vi "SysDef.Node.Info.vi"(8 "error in (no error)":errorcluster, 11 "nodeID":u64) -> (0 "error out":errorcluster, 1 "Item Info":T1, 3 "nodeID out":u64, 4 "Found?":bool)   [LabVIEW 2019, in "Advanced System Definition.lvlib"]
uses:
  Advanced System Definition.lvlib
  _Types/TreeItem.Info.ctl
  <vilib>/NI VeriStand/Custom Device API/Custom Device Channel.ctl
  <vilib>/NI VeriStand/Custom Device API/Custom Device Channel Type.ctl
  <vilib>/NI VeriStand/Custom Device API/Custom Device Waveform.ctl
  <vilib>/NI VeriStand/Custom Device API/Custom Device Waveform DataType.ctl
  NationalInstruments.VeriStand.SystemDefinitionAPI
  <vilib>/NI VeriStand/Custom Device API/Custom Device API.lvlib
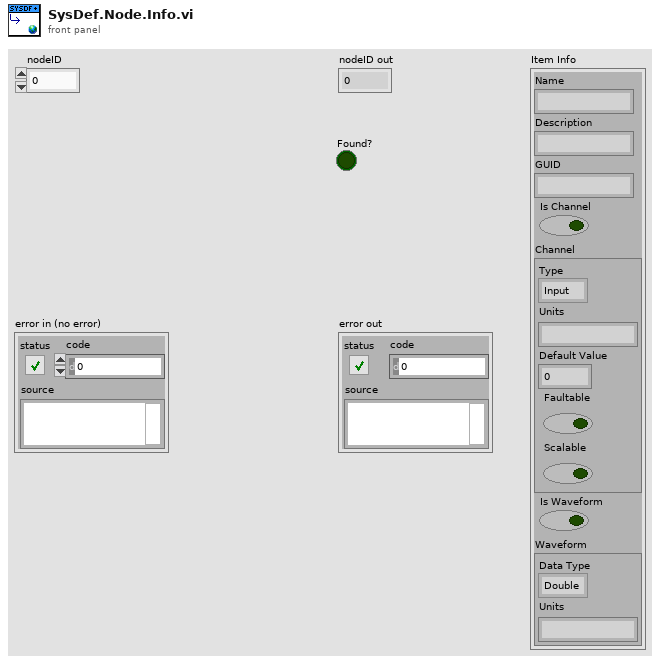
[diagram p1: front panel]
types:
  T1 = typedef "Advanced System Definition.lvlib/TreeItem.Info.ctl" = cluster{"Name":string, "Description":string, "GUID":string, "Is Channel":bool, "Channel":T2, "Is Waveform":bool, "Waveform":T4}
  T2 = typedef "Custom Device API.lvlib/Custom Device Channel.ctl" = cluster{"Type":T3, "Units":string, "Default Value":dbl, "Faultable":bool, "Scalable":bool}
  T3 = typedef "Custom Device API.lvlib/Custom Device Channel Type.ctl" = enum16{"Input", "Output"}
  T4 = typedef "Custom Device API.lvlib/Custom Device Waveform.ctl" = cluster{"Data Type":T5, "Units":string}
  T5 = typedef "Custom Device API.lvlib/Custom Device Waveform DataType.ctl" = enum16{"Double", "Complex Double"}
  T6 = typedef "Custom Device API.lvlib/Custom Device Item Info.ctl" = cluster{"Name":string, "Is Channel":bool, "GUID":string, "Is Waveform":bool}
  T7 = typedef "Custom Device API.lvlib/Custom Device Item Ref.ctl" = u64
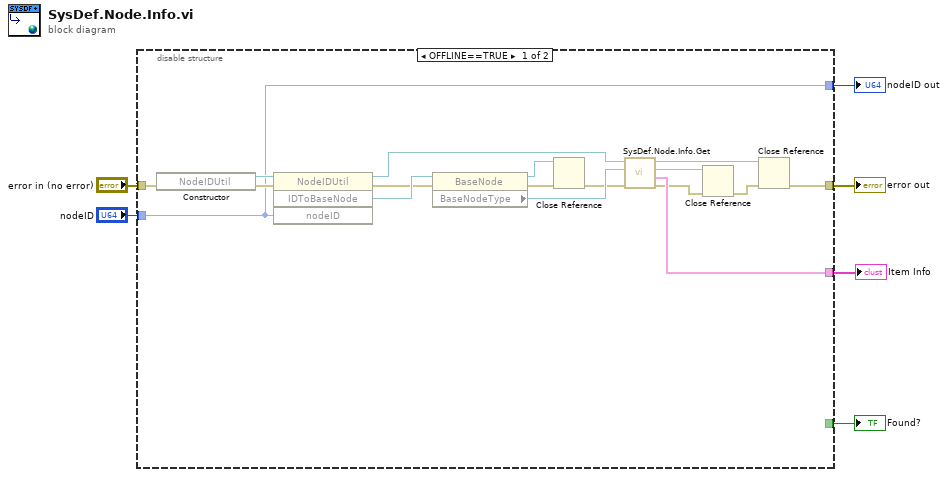
[diagram p0: block diagram]
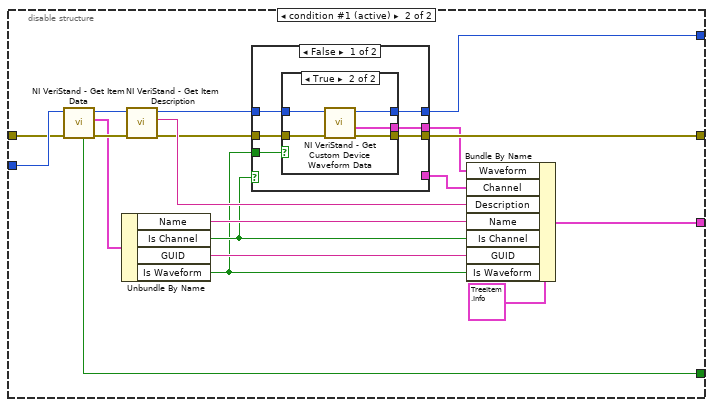
[diagram p2: hidden frame]
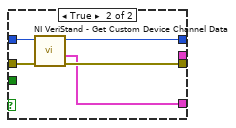
[diagram p4: hidden frame]
diagram:
  n1 = disable-structure shown="OFFLINE==TRUE" {
    disable-tunnel: "error in (no error)" -> [w20 w41]
    disable-tunnel: "nodeID" -> [w16 w42]
    disable-tunnel: [w17 w26] -> w4
    disable-tunnel: [_ w40] -> w3
    disable-tunnel: [w13 w32] -> w2
    disable-tunnel: [w16 w25] -> w1
    frame condition #0 {
      n2 = constructor class="NodeIDUtil"(error in=w20) -> (reference out=w23:refnum<k24>, error out=w22:errorcluster)  [unwired: 2 in, 1 out]
      n3 = invoke class="NodeIDUtil" method="IDToBaseNode"(reference=w23, error in=w22, "nodeID"=w16) -> (reference out=w9:refnum<k24>, error out=w7:errorcluster, "IDToBaseNode"=w21:refnum<k24>)  [unwired: 1 in, 1 out]
      n4 = property class="BaseNode"(reference=w21, error in=w7) -> (reference out=w19:refnum<k24>, error out=w18:errorcluster, "BaseNodeType"=w14:refnum<k24>)
      n5 = Close Reference(reference=w19, error in (no error)=w18) -> (error out=w8:errorcluster)
      n6 = call "SysDef.Node.Info.Get.vi"("error in (no error)"=w8, "BaseNode Ref"=w14, "NodeIDUtil Ref in"=w9) -> ("error out"=w11:errorcluster, "Item Info"=w13:T1, "BaseNode Ref out"=w12:refnum<k24>, "NodeIDUtil Ref out"=w10:refnum<k24>)  [unwired: 5 in]
      n7 = Close Reference(reference=w12, error in (no error)=w11) -> (error out=w15:errorcluster)
      n8 = Close Reference(reference=w10, error in (no error)=w15) -> (error out=w17:errorcluster)
    }
    frame condition #1 (active) {
      n9 = call <vilib>:"NI VeriStand - Get Item Data.vi"("error in (no error)"=w41, "Item Ref in"=w42) -> ("error out"=w35:errorcluster, "Item Info"=w33:T6, "Item Ref out"=w36:T7, "Found"=w40:bool)  [unwired: 6 in]
      n10 = Unbundle By Name(w33) -> ("Name"=w38:string, "Is Channel"=w31:bool, "GUID"=w37:string, "Is Waveform"=w28:bool)
      n11 = call <vilib>:"NI VeriStand - Get Item Description.vi"("error in (no error)"=w35, "Item Ref in"=w36) -> ("error out"=w30:errorcluster, "Description"=w34:string, "Item Ref out"=w29:T7)  [unwired: 6 in, 1 out]
      n12 = case shown="False" w31 {
        tunnel: w30 -> [w47 w60]
        tunnel: w29 -> [w46 w59]
        tunnel: w28 -> [w48 _]
        tunnel: [w45 w58] -> w26
        tunnel: [_ w57] -> w27
        tunnel: [w44 w56] -> w25
        tunnel: [w43 _] -> w24
        frame False {
          n13 = case shown="True" w48 {
            tunnel: w47 -> [w50 w55]
            tunnel: w46 -> [w49 w54]
            tunnel: [w50 w53] -> w45
            tunnel: [w49 w52] -> w44
            tunnel: [_ w51] -> w43
            frame False {
            }
            frame True {
              n14 = call <vilib>:"NI VeriStand - Get Custom Device Waveform Data.vi"("error in (no error)"=w55, "Waveform Ref in"=w54) -> ("error out"=w53:errorcluster, "Waveform"=w51:T4, "Waveform Ref out"=w52:T7)  [unwired: 4 in, 3 out]
            }
          }
        }
        frame True {
          n15 = call <vilib>:"NI VeriStand - Get Custom Device Channel Data.vi"("error in (no error)"=w60, "Channel Ref in"=w59) -> ("error out"=w58:errorcluster, "Channel"=w57:T2, "Channel Ref out"=w56:T7)  [unwired: 4 in, 3 out]
        }
      }
      n16 = Bundle By Name(cluster=T1 {"Name"="", "Description"="", "GUID"="", "Is Channel"=FALSE, "Channel"={"Type"=enum."Input", "Units"="", "Default Value"=0.0, "Faultable"=FALSE, "Scalable"=FALSE}, "Is Waveform"=FALSE, "Waveform"={"Data Type"=enum."Double", "Units"=""}} ("Item Info"), "Waveform"=w24, "Channel"=w27, "Description"=w34, "Name"=w38, "Is Channel"=w31, "GUID"=w37, "Is Waveform"=w28) -> (w32:T1)
    }
  }
  "nodeID out" <- w1
  "error out" <- w4
  "Item Info" <- w2
  "Found?" <- w3
